vi "sort_Controls_Column.vi"(10 "Controls":refnum<vi>[](array[refnum]), 11 "Area Scale":T1) -> ()   [LabVIEW 2015]
uses:
  <vilib>/Utility/miscctls.llb/LVRectTypeDef.ctl
panel:
  in  "Index":i32
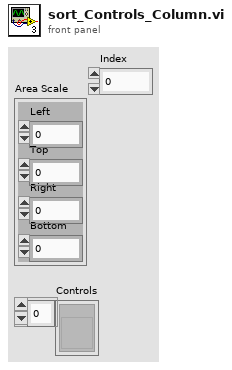
[diagram p1: front panel]
types:
  T1 = typedef "LVRectTypeDef.ctl" = cluster{"Left":i16, "Top":i16, "Right":i16, "Bottom":i16}
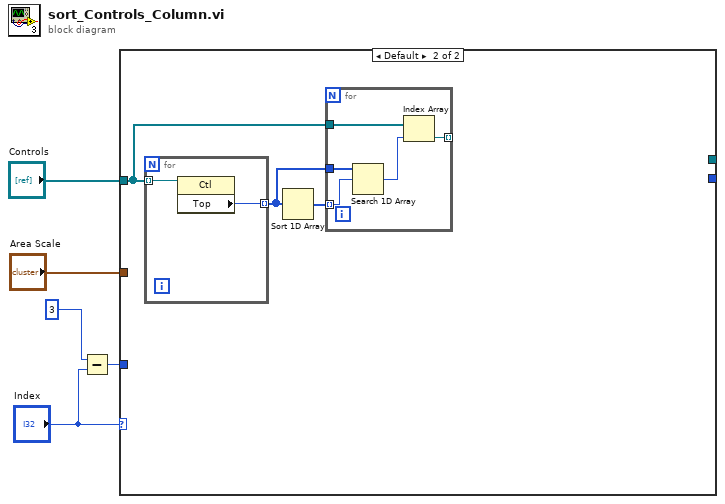
[diagram p0: block diagram]
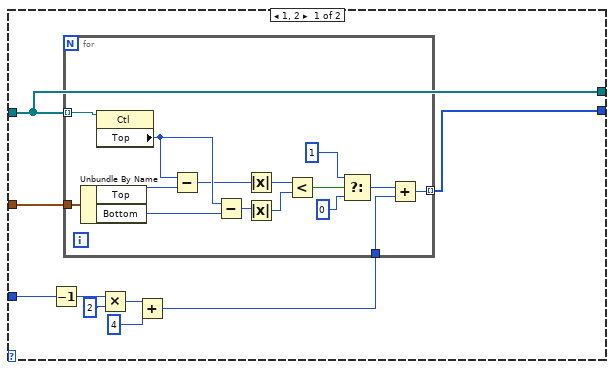
[diagram p2: hidden frame]
diagram:
  n1 = Subtract(x=3, y="Index") -> (x-y=w1:i32)
  n2 = case shown="Default" "Index" {
    tunnel: "Controls" -> [w9 w30]
    tunnel: "Area Scale" -> [w8 _]
    tunnel: w1 -> [w14 _]
    tunnel: [w9 _] -> _
    tunnel: [w6 _] -> _
    frame 1, 2 {
      n3 = Decrement(x=w14) -> (x-1=w13:i32)
      n4 = Multiply(x=w13, y=2) -> (x*y=w11:i32)
      n5 = Add(x=w11, y=4) -> (x+y=w7:i32)
      n6 = for {
        tunnel: w9 -> [w29] mode=indexing
        tunnel: w8 -> [w28]
        tunnel: w7 -> [w16]
        tunnel: [w15] -> w6 mode=indexing
        n7 = Unbundle By Name(w28) -> ("Top"=w27:i16, "Bottom"=w25:i16)
        n8 = property class="Ctl"(reference=w29) -> ("Top"=w26:i32)  [unwired: 1 in, 2 out]
        n9 = Subtract(x=w26, y=w27) -> (x-y=w24:i32)
        n10 = Subtract(x=w26, y=w25) -> (x-y=w23:i32)
        n11 = Absolute Value(x=w24) -> (abs(x)=w22:i32)
        n12 = Absolute Value(x=w23) -> (abs(x)=w21:i32)
        n13 = Less?(x=w22, y=w21) -> (x < y?=w20:bool)
        n14 = Select(t=1, s=w20, f=0) -> (s? t:f=w17:i32)
        n15 = Add(x=w17, y=w16) -> (x+y=w15:i32)
      }
    }
    frame Default {
      n16 = for {
        tunnel: w30 -> [w39] mode=indexing
        tunnel: [w38] -> w31 mode=indexing
        n17 = property class="Ctl"(reference=w39) -> ("Top"=w38:i32)  [unwired: 1 in, 2 out]
      }
      n18 = Sort 1D Array(array=w31) -> (sorted array=w32:i32[])
      n19 = for {
        tunnel: w32 -> [w36] mode=indexing
        tunnel: w31 -> [w37]
        tunnel: w30 -> [w35]
        tunnel: [w33] -> _ mode=indexing
        n20 = Search 1D Array(1D array=w37, element=w36) -> (index of element=w34:i32)  [unwired: 1 in]
        n21 = Index Array(array=w35, index=w34) -> (element=w33:refnum<vi>)
      }
    }
  }
